vi "Write Sequential Address.vi"(7 "BCI-1553 Device":refnum<k21>, 8 "Data 3":u16, 9 "Data 2":u16, 10 "Data 1":u16, 11 "Command":u8) -> ()   [LabVIEW 2020, in "BCI-1553 RT Interface.lvlib"]
doc: "Performs sequential address writing."
uses:
  BCI-1553 RT Interface.lvlib
  <vilib>/rvi/eio/common/nirviEmuTemplateMethod_errors.vi
  <vilib>/eio/EIOMethodNode/EIOMethodNode.xnode
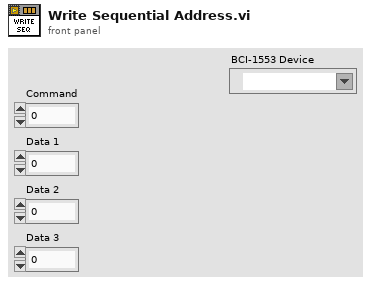
[diagram p1: front panel]
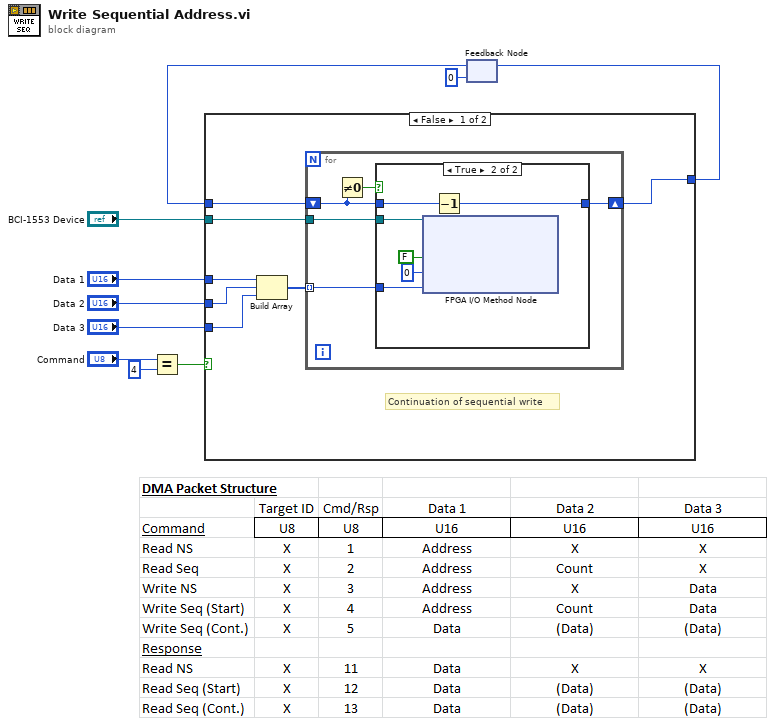
[diagram p0: block diagram]
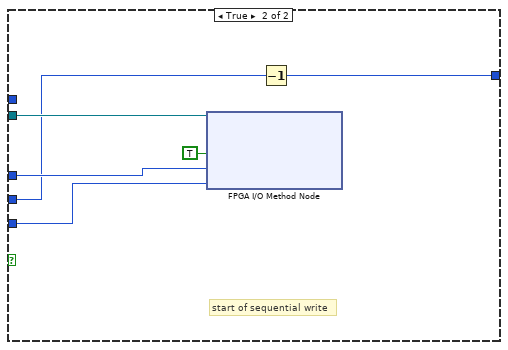
[diagram p3: hidden frame]
diagram:
  n1 = Equal?(x="Command", y=u8 4) -> (x = y?=w8:bool)
  n2 = feedback #1(u16 0 ("Data 2")) -> (w1:u16)
  n3 = case shown="False" w8 {
    tunnel: "Data 1" -> [w17 w33]
    tunnel: "Data 2" -> [w16 w31]
    tunnel: "Data 3" -> [w15 w32]
    tunnel: "BCI-1553 Device" -> [w13 w35]
    tunnel: [w11 w30] -> w2
    tunnel: w1 -> [w12 _]
    frame False {
      # "Continuation of sequential write"
      n4 = Build Array(w17, w16, w15) -> (w14:u16[])
      n5 = for {
        tunnel: w14 -> [w18] mode=indexing
        tunnel: w13 -> [w19]
        shift-right: [w20] -> w11
        shift-left: w12 -> [w21]
        n6 = Not Equal To 0?(x=w21) -> (x != 0?=w22:bool)
        n7 = case shown="True" w22 {
          tunnel: w21 -> [w23 w29]
          tunnel: [w23 w28] -> w20
          tunnel: w19 -> [_ w27]
          tunnel: w18 -> [_ w25]
          frame False {
          }
          frame True {
            n8 = xnode "FPGA I/O Method Node"("FPGA I/O In"=w27, "Initialize"=FALSE, "Address"=u16 0, "Data"=w25) -> ()  [unwired: 1 out]
            n9 = Decrement(x=w29) -> (x-1=w28:u16)
          }
        }
      }
    }
    frame True {
      # "start of sequential write"
      n10 = xnode "FPGA I/O Method Node"("FPGA I/O In"=w35, "Initialize"=TRUE, "Address"=w33, "Data"=w32) -> ()  [unwired: 1 out]
      n11 = Decrement(x=w31) -> (x-1=w30:u16)
    }
  }
  n12 = feedback-in #1(w2) -> ()
